vi "InitSimulation.vi"(6 "Instance":i32, 8 "error in (no error)":errorcluster, 11 "Simulation Data":T1={"plenght"=50.0, "cartMass"=10.0, "pendulumMass"=10.0, "angle"=0.0}) -> (0 "error out":errorcluster)   [LabVIEW 2017, in "PendulumLoop.lvlib"]
uses:
  PendulumLoop.lvlib
  Communication/Communication.lvlib
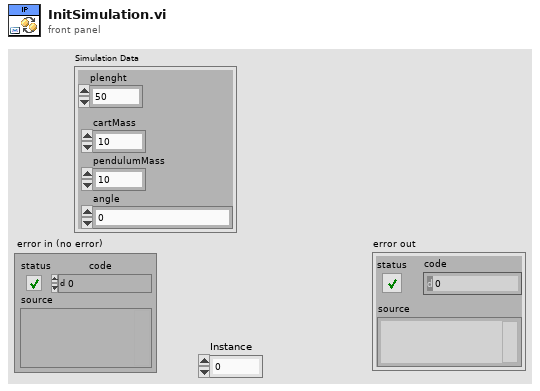
[diagram p1: front panel]
types:
  T1 = cluster{"plenght":dbl, "cartMass":dbl, "pendulumMass":dbl, "angle":dbl}
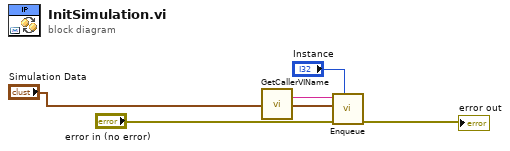
[diagram p0: block diagram]
diagram:
  n1 = call "GetCallerVIName.vi"() -> ("VI name"=w2:string)  [unwired: 11 in]
  n2 = call "Enqueue.vi"("Instance"="Instance", "error in (no error)"="error in (no error)", "Data"="Simulation Data", "Msg"=w2) -> ("error out"=→"error out":errorcluster)  [unwired: 7 in]
